vi "Open.vi"(8 "error in (no error)":errorcluster, 10 "Channel Names":tag[](array[tag])) -> (0 "error out":errorcluster, 3 "AO (Continuous) Ref Out":T1)   [LabVIEW 2021, in "AO Continuous.lvlib"]
uses:
  <vilib>/myRIO/Instrument Drivers/Onboard IO/AO Continuous/AO Continuous.lvlib
  <vilib>/myRIO/Instrument Drivers/Onboard IO/AO Continuous/typedefs/AO Continuous Reference.ctl
  <vilib>/myRIO/Common/Instrument Driver Framework/Utilities/typedefs/myRIO Generic Hardware Reference.ctl
  <vilib>/myRIO/Common/Instrument Driver Framework/Utilities/typedefs/Hardware Version Enum.ctl
  <vilib>/myRIO/Common/Instrument Driver Framework/Utilities/typedefs/myRIO v1.0 Reference.ctl
  <vilib>/myRIO/Common/Instrument Driver Framework/Utilities/typedefs/Generic FPGA Reference.ctl
  <vilib>/myRIO/Common/Instrument Driver Framework/ELVIS III v1.0/AO Continuous/typedefs/AO Continuous Channels List.ctl
  <vilib>/myRIO/Common/Instrument Driver Framework/ELVIS III v1.0/AO Continuous/typedefs/ELVIS III v1.0 AO Continuous Channels Enum.ctl
  <vilib>/myRIO/Common/Instrument Driver Framework/ELVIS III v1.0/AO Continuous/typedefs/AO Continuous Channel Info.ctl
  <vilib>/userdefined/High Color/nirio_resource_hc.ctl
panel:
  # "AO (Continuous) Open"
  # "Opens a reference to the myRIO hardware and configures the AO Continuous Reference with channels to be read"
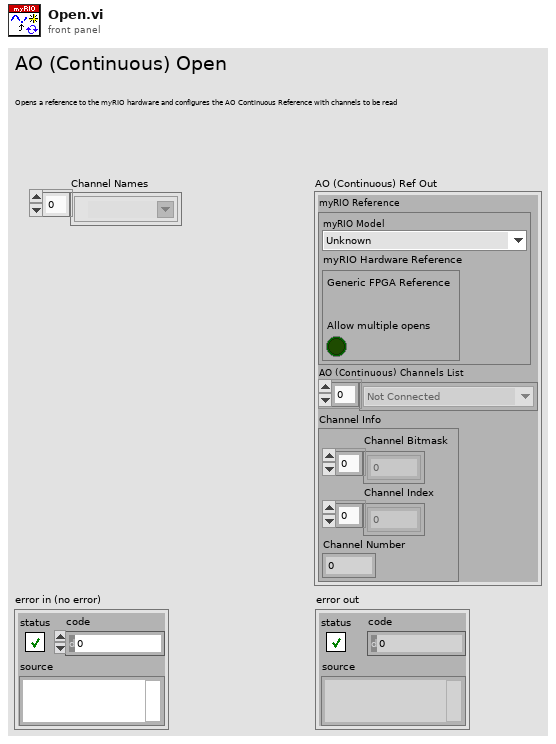
[diagram p1: front panel]
types:
  T1 = typedef "AO Continuous.lvlib/AO Continuous Reference.ctl" = cluster{"myRIO Reference":T2, "AO (Continuous) Channels List":T6, "Channel Info":T8}
  T2 = typedef "myRIO Generic Hardware Reference.ctl" = cluster{"myRIO Model":T3, "myRIO Hardware Reference":T4}
  T3 = typedef "Hardware Version Enum.ctl" = enum16{"Unknown", "myRIO-1900", "myRIO-1950", "roboRIO", "NI ELVIS RIO CM", "ELVIS III"}
  T4 = typedef "myRIO v1.0 Reference.ctl" = cluster{"Generic FPGA Reference":T5, "Allow multiple opens":bool}
  T5 = typedef "Generic FPGA Reference.ctl" = refnum<k20>
  T6 = typedef "AO Continuous Channels List.ctl" = T7[]
  T7 = typedef "ELVIS III v1.0 AO Continuous Channels Enum.ctl" = enum16{"Not Connected", "A/AO0 (Continuous)", "A/AO1 (Continuous)", "B/AO0 (Continuous)", "B/AO1 (Continuous)"}
  T8 = typedef "AO Continuous Channel Info.ctl" = cluster{"Channel Bitmask":u8[], "Channel Index":i32[], "Channel Number":u8}
  T9 = typedef "nirio_resource_hc.ctl" = tag
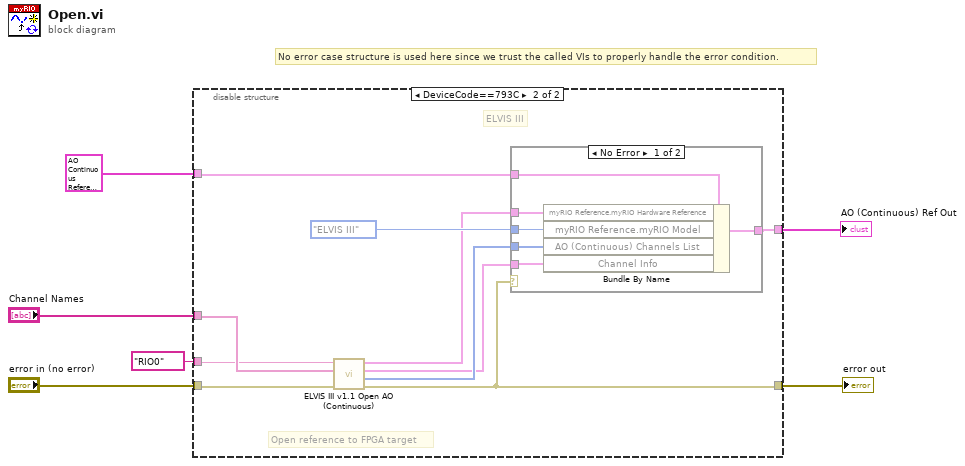
[diagram p0: block diagram]
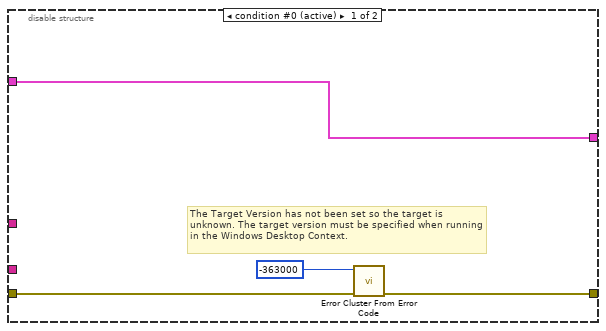
[diagram p2: hidden frame]
diagram:
  # "No error case structure is used here since we trust the called VIs to properly handle the error condition."
  n1 = disable-structure shown="DeviceCode==793C" {
    disable-tunnel: [w10 w12] -> w5
    disable-tunnel: "Channel Names" -> [_ w15]
    disable-tunnel: [w7 w11] -> w4
    disable-tunnel: "error in (no error)" -> [w9 w13]
    disable-tunnel: T1 {"myRIO Reference"={"myRIO Model"=enum."Unknown", "myRIO Hardware Reference"={"Generic FPGA Reference"=refnum, "Allow multiple opens"=FALSE}}, "AO (Continuous) Channels List"=[], "Channel Info"={"Channel Bitmask"=[], "Channel Index"=[], "Channel Number"=0}} ("AO (N Samples) Write Ref Out") -> [w7 w16]
    disable-tunnel: T9 "RIO0" ("Resource name") -> [_ w14]
    frame condition #0 (active) {
      # "The Target Version has not been set so the target is unknown. The target version must be specified when running in the Windows Desktop Context."
      n2 = call <vilib>:"Error Cluster From Error Code.vi"("error in (no error)"=w9, "error code (0)"=-363000) -> ("error out"=w10:errorcluster)  [unwired: 7 in]
    }
    frame condition #1 {
      # "ELVIS III"
      # "Open reference to FPGA target"
      n3 = call <vilib>:"ELVIS III v1.1 Open AO (Continuous).vi"("error in (no error)"=w13, "Channel Names"=w15, "Resource name"=w14) -> ("error out"=w12:errorcluster, "AO (Continuous) Channels List"=w18:T6, "Channel Info"=w17:T8, "AO (Continuous) Ref Out"=w19:T4)  [unwired: 5 in]
      n4 = case shown="No Error" w12 {
        tunnel: [w26 w27] -> w11
        tunnel: Hardware_Version_Enum."ELVIS III" ("Hardware Version Enum") -> [w25 _]
        tunnel: w16 -> [w24 w27]
        tunnel: w19 -> [w23 _]
        tunnel: w18 -> [w22 _]
        tunnel: w17 -> [w21 _]
        frame No Error {
          n5 = Bundle By Name(cluster=w24, "myRIO Reference.myRIO Hardware Reference"=w23, "myRIO Reference.myRIO Model"=w25, "AO (Continuous) Channels List"=w22, "Channel Info"=w21) -> (w26:T1)
        }
        frame Error {
        }
      }
    }
  }
  "AO (Continuous) Ref Out" <- w4
  "error out" <- w5
